vi "SmartInsert.vi"(8 "error in (no error)":errorcluster, 10 "VI reference In":refnum<vi>, 11 "SelList[]":refnum<vi>[](array[refnum])) -> (0 "error out":errorcluster)   [LabVIEW 2014]
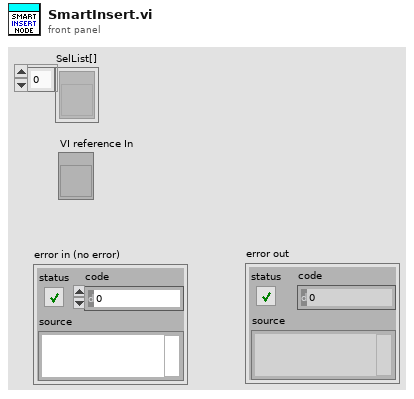
[diagram p1: front panel]
types:
  T1 = cluster{"Source":refnum<vi>, "Sink":refnum<vi>, "Type Variant":variant}
  T2 = typedef "LVPositionTypeDef.ctl" = cluster{"Left":i32, "Top":i32}
  T3 = cluster{"Position":cluster{"h":i16, "v":i16}, "Flags":i32, "Type":enum32{"LooseEnd", "Endpoint", "Bend", "Junction"}, "Up Joint Index":i16, "Down Joint Index":i16, "Left Joint Index":i16, "Right Joint Index":i16}[]
  T4 = typedef "LVPointTypeDef.ctl" = cluster{"Horizontal":i16, "Vertical":i16}
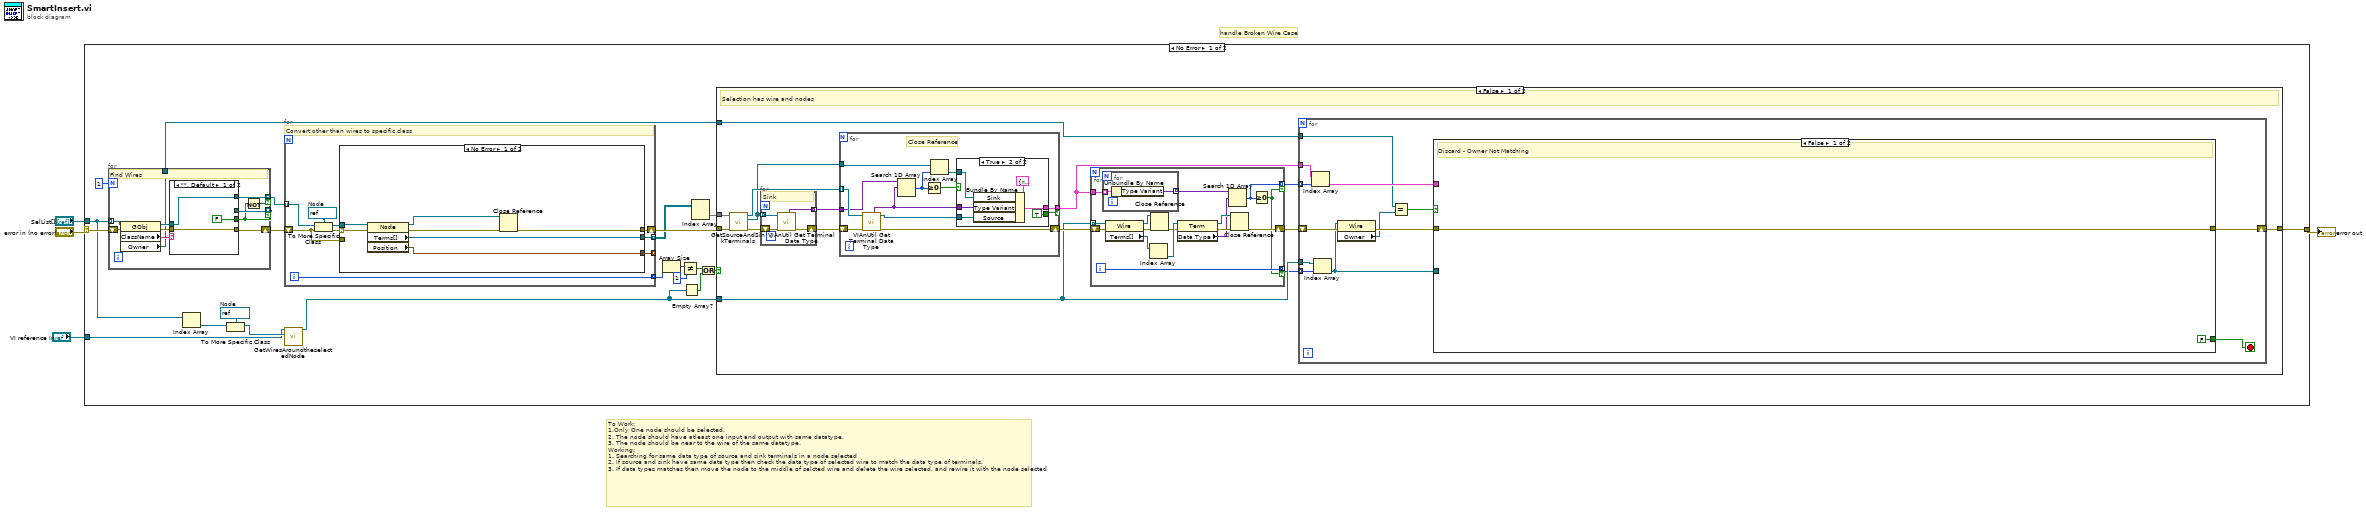
[diagram p0: block diagram]
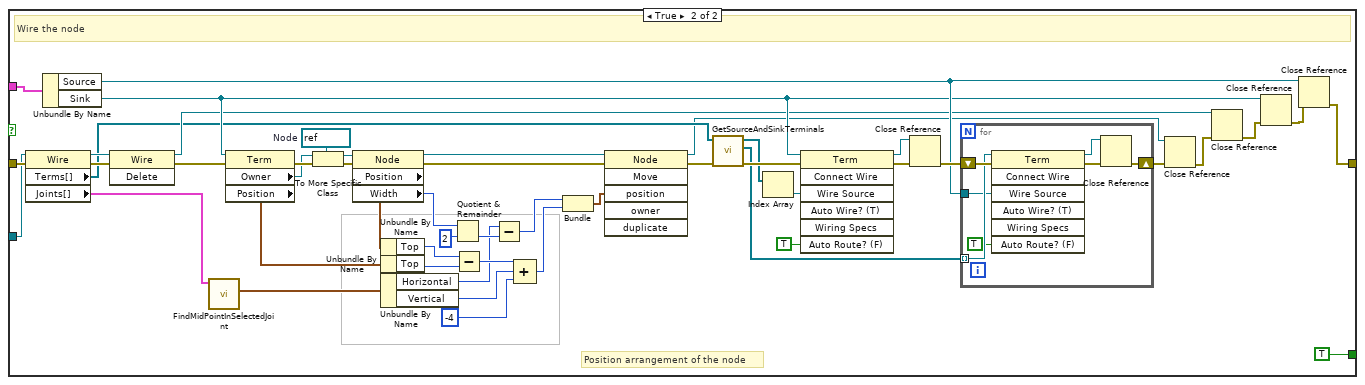
[diagram p2: hidden frame]
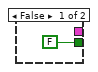
[diagram p3: hidden frame]
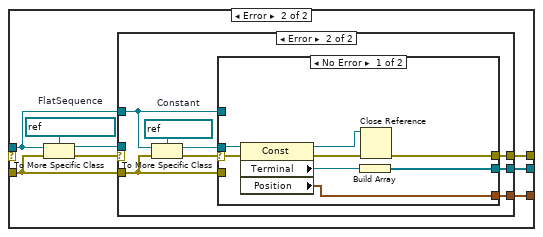
[diagram p5: hidden frame]
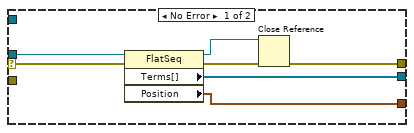
[diagram p6: hidden frame]
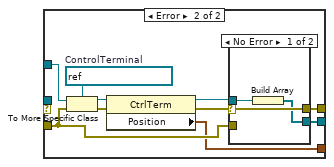
[diagram p7: hidden frame]
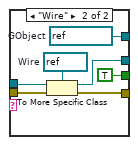
[diagram p9: hidden frame]
diagram:
  # "To Work:\n1.Only One node should be selected.\n2. The node should have atleast one input and output with same datatype.\n3. The node should be near to the wire of the same datatype.\nWorking:\n1. Searching for same data type of source and sink terminals in a node selected\n2. If source and sink have same data type then check the data type of selected wire to match the data type of terminals.\n3. If data types matches then move the node to the middle of selcted wire and delete the wire selected, and rewire it with the node selected"
  # "handle Broken Wire Case"
  n1 = case shown="No Error" "error in (no error)" {
    selector: "error in (no error)" -> [w25 w236]
    tunnel: [w21 w236] -> w2
    tunnel: "SelList[]" -> [w11 _]
    tunnel: "VI reference In" -> [w8 _]
    frame No Error {
      w12 = refnum<vi> refnum  # Node
      n2 = for {
        N: 1 -> [_]
        tunnel: w11 -> [w225] mode=indexing
        tunnel: [w219] -> _ mode=indexing if=w217
        shift-right: [w220] -> w24
        shift-left: w25 -> [w222]
        tunnel: [w218] -> w23 mode=indexing if=w216
        tunnel: [w215] -> w5
        # "Find Wires"
        n3 = property on="Property Node" class="GObj"(reference=w225, error in=w222) -> (reference out=w223:refnum<vi>, error out=w221:errorcluster, "ClassName"=w224:string, "Owner"=w215:refnum<vi>)
        n4 = case shown="\"\", Default" w224 {
          tunnel: w223 -> [w226 w233]
          tunnel: w221 -> [w227 w235]
          tunnel: [w227 w234] -> w220
          tunnel: [_ w231] -> w219
          tunnel: [FALSE TRUE] -> w217
          tunnel: [w226 w229] -> w218
          frame "", Default {
          }
          frame "Wire" {
            w229 = refnum<vi> refnum  # GObject
            w232 = refnum<vi> refnum  # Wire
            n5 = To More Specific Class(target class=w232, reference=w233, error in=w235) -> (specific class reference=w231:refnum<vi>, error out=w234:errorcluster)
          }
        }
        n6 = Not(x=w217) -> (.not. x?=w216:bool)
      }
      n7 = Index Array(array=w11) -> (element=w10:refnum<vi>)  [unwired: 1 in]
      n8 = To More Specific Class(target class=w12, reference=w10) -> (specific class reference=w9:refnum<vi>)  [unwired: 1 in, 1 out]
      n9 = for {
        tunnel: [w160] -> w20 mode=indexing
        shift-right: [w157] -> w22
        shift-left: w24 -> [w158]
        tunnel: w23 -> [w156] mode=indexing
        tunnel: [w155] -> w17 mode=indexing
        tunnel: [w154] -> _ mode=indexing
        i -> [w155]
        w159 = refnum<vi> refnum  # Node
        # "Convert other than wires to specific class"
        n10 = To More Specific Class(target class=w159, reference=w156, error in=w158) -> (specific class reference=w161:refnum<vi>, error out=w162:errorcluster)
        n11 = case shown="No Error" w162 {
          selector: w162 -> [w169 _]
          tunnel: w161 -> [w168 w171]
          tunnel: [w167 w173] -> w160
          tunnel: [w165 w175] -> w157
          tunnel: w158 -> [_ w174]
          tunnel: [w163 w170] -> w154
          frame No Error {
            n12 = property on="Property Node" class="Node"(reference=w168, error in=w169) -> (reference out=w164:refnum<vi>, error out=w166:errorcluster, "Terms[]"=w167:refnum<vi>[], "Position"=w163:T2)
            n13 = Close Reference(reference=w164, error in (no error)=w166) -> (error out=w165:errorcluster)
          }
          frame Error {
            w172 = refnum<vi> refnum  # FlatSequence
            n14 = To More Specific Class(target class=w172, reference=w171, error in=w174) -> (specific class reference=w176:refnum<vi>, error out=w177:errorcluster)
            n15 = case shown="Error" w177 {
              selector: w177 -> [w184 _]
              tunnel: w176 -> [w183 _]
              tunnel: [w180 w187] -> w175
              tunnel: w174 -> [_ w189]
              tunnel: [w181 w188] -> w173
              tunnel: w171 -> [_ w190]
              tunnel: [w178 w185] -> w170
              frame No Error {
                n16 = property on="Property Node" class="FlatSeq"(reference=w183, error in=w184) -> (reference out=w179:refnum<vi>, error out=w182:errorcluster, "Terms[]"=w181:refnum<vi>[], "Position"=w178:T2)
                n17 = Close Reference(reference=w179, error in (no error)=w182) -> (error out=w180:errorcluster)
              }
              frame Error {
                w186 = refnum<vi> refnum  # Constant
                n18 = To More Specific Class(target class=w186, reference=w190, error in=w189) -> (specific class reference=w191:refnum<vi>, error out=w192:errorcluster)
                n19 = case shown="No Error" w192 {
                  selector: w192 -> [w199 _]
                  tunnel: w191 -> [w200 _]
                  tunnel: w190 -> [_ w210]
                  tunnel: w189 -> [_ w208]
                  tunnel: [w197 w206] -> w188
                  tunnel: [w195 w207] -> w187
                  tunnel: [w193 w201] -> w185
                  frame No Error {
                    n20 = property on="Property Node" class="Const"(reference=w200, error in=w199) -> (reference out=w194:refnum<vi>, error out=w196:errorcluster, "Terminal"=w198:refnum<vi>, "Position"=w193:T2)
                    n21 = Build Array(w198) -> (w197:refnum<vi>[])
                    n22 = Close Reference(reference=w194, error in (no error)=w196) -> (error out=w195:errorcluster)
                  }
                  frame Error {
                    w205 = refnum<vi> refnum  # ControlTerminal
                    n23 = To More Specific Class(target class=w205, reference=w210, error in=w208) -> (specific class reference=w203:refnum<vi>, error out=w209:errorcluster)
                    n24 = property class="CtrlTerm"(reference=w203, error in=w209) -> (reference out=w202:refnum<vi>, error out=w204:errorcluster, "Position"=w201:T2)
                    n25 = case shown="No Error" w204 {
                      selector: w204 -> [w213 _]
                      tunnel: w202 -> [w212 _]
                      tunnel: w208 -> [_ w214]
                      tunnel: [w213 w214] -> w207
                      tunnel: [w211 _] -> w206
                      frame No Error {
                        n26 = Build Array(w212) -> (w211:refnum<vi>[])
                      }
                      frame Error {
                      }
                    }
                  }
                }
              }
            }
          }
        }
      }
      n27 = call "GetWiresAroundtheselectedNode.vi"("Sel Node reference"=w9, "VI reference In"=w8) -> ("WiresInRange[]"=w7:refnum<vi>[])  [unwired: 8 in, 1 out]
      n28 = Array Size(array=w17) -> (size(s)=w19:i32)
      n29 = Not Equal?(x=w19, y=1) -> (x != y?=w15:bool)
      n30 = Empty Array?(array=w7) -> (empty?=w14:bool)
      n31 = Index Array(array=w20) -> (element=w18:refnum<vi>[])  [unwired: 2 in]
      n32 = Or(x=w15, y=w14) -> (x .or. y?=w13:bool)
      n33 = case shown="False" w13 {
        tunnel: w7 -> [w32 _]
        tunnel: [w34 w153] -> w21
        tunnel: w22 -> [w40 w153]
        tunnel: w18 -> [w27 _]
        tunnel: w5 -> [w26 _]
        frame False {
          # "Selection has wire and nodes"
          n34 = call "GetSourceAndSinkTerminals.vi"("error in (no error)"=w40, "Terms[]"=w27) -> ("error out"=w38:errorcluster, "Sink"=w28:refnum<vi>[], "Source"=w36:refnum<vi>[])  [unwired: 7 in]
          n35 = for {
            tunnel: w28 -> [w133] mode=indexing
            tunnel: [w132] -> w39 mode=indexing
            shift-right: [w130] -> w37
            shift-left: w38 -> [w131]
            # "Sink"
            n36 = call <vilib>:"VIAnUtil Get Terminal Data Type.vi"("error in (no error)"=w131, "Terminal"=w133) -> ("error out"=w130:errorcluster, "Type Variant"=w132:variant)  [unwired: 6 in, 2 out]
          }
          n37 = for {
            tunnel: w39 -> [w144]
            tunnel: w36 -> [w145] mode=indexing
            shift-right: [w141] -> w35
            shift-left: w37 -> [w142]
            tunnel: w28 -> [w138]
            tunnel: [w135] -> w30 mode=indexing if=w134
            # "Close Reference"
            n38 = call <vilib>:"VIAnUtil Get Terminal Data Type.vi"("error in (no error)"=w142, "Terminal"=w145) -> ("error out"=w141:errorcluster, "dup  Terminal"=w140:refnum<vi>, "Type Variant"=w143:variant)  [unwired: 6 in, 1 out]
            n39 = Search 1D Array(1D array=w144, element=w143) -> (index of element=w139:i32)  [unwired: 1 in]
            n40 = Greater Or Equal To 0?(x=w139) -> (x >= 0?=w136:bool)
            n41 = Index Array(array=w138, index=w139) -> (element=w137:refnum<vi>)
            n42 = case shown="True" w136 {
              tunnel: w143 -> [_ w151]
              tunnel: w140 -> [_ w150]
              tunnel: w137 -> [_ w149]
              tunnel: [_ w148] -> w135
              tunnel: [FALSE TRUE] -> w134
              frame False {
              }
              frame True {
                n43 = Bundle By Name(cluster=T1 {"Source"=refnum, "Sink"=refnum, "Type Variant"=variant}, "Sink"=w149, "Type Variant"=w151, "Source"=w150) -> (w148:T1)
              }
            }
          }
          n44 = for {
            tunnel: w32 -> [w125] mode=indexing
            shift-right: [w121] -> w33
            shift-left: w35 -> [w127]
            tunnel: w30 -> [w119]
            tunnel: [w116] -> w29 mode=indexing if=w112
            tunnel: [w115] -> w31 mode=indexing if=w112
            i -> [w115]
            n45 = for {
              tunnel: w119 -> [w129] mode=indexing
              tunnel: [w128] -> w118 mode=indexing
              n46 = Unbundle By Name(w129) -> ("Type Variant"=w128:variant)
            }
            n47 = property on="Property Node" class="Wire"(reference=w125, error in=w127) -> (reference out=w113:refnum<vi>, error out=w126:errorcluster, "Terms[]"=w124:refnum<vi>[])
            n48 = Index Array(array=w124) -> (element=w122:refnum<vi>)  [unwired: 1 in]
            n49 = Close Reference(reference=w113, error in (no error)=w126) -> (error out=w114:errorcluster)
            n50 = property on="Property Node" class="Term"(reference=w122, error in=w114) -> (reference out=w120:refnum<vi>, error out=w123:errorcluster, "Data Type"=w117:variant)
            n51 = Search 1D Array(1D array=w118, element=w117) -> (index of element=w116:i32)  [unwired: 1 in]
            n52 = Close Reference(reference=w120, error in (no error)=w123) -> (error out=w121:errorcluster)
            n53 = Greater Or Equal To 0?(x=w116) -> (x >= 0?=w112:bool)
          }
          n54 = for {
            tunnel: w32 -> [w51]
            tunnel: w31 -> [w50] mode=indexing
            tunnel: w30 -> [w49]
            tunnel: w29 -> [w47] mode=indexing
            shift-right: [w53] -> w34
            shift-left: w33 -> [w52]
            tunnel: w26 -> [w42]
            stop <- w46 stop-if-true
            n55 = Index Array(array=w49, index=w47) -> (element=w48:T1)
            n56 = Index Array(array=w51, index=w50) -> (element=w44:refnum<vi>)
            n57 = property class="Wire"(reference=w44, error in=w52) -> (error out=w45:errorcluster, "Owner"=w43:refnum<vi>)  [unwired: 1 out]
            n58 = Equal?(x=w42, y=w43) -> (x = y?=w41:bool)
            n59 = case shown="False" w41 {
              tunnel: [w55 w95] -> w53
              tunnel: w45 -> [w55 w104]
              tunnel: w48 -> [_ w58]
              tunnel: w44 -> [_ w57]
              tunnel: [FALSE TRUE] -> w46
              frame False {
                # "Discard - Owner Not Matching"
              }
              frame True {
                w87 = refnum<vi> refnum  # Node
                # "Position arrangement of the node"
                # "Wire the node"
                n60 = property on="Property Node" class="Wire"(reference=w57, error in=w104) -> (reference out=w91:refnum<vi>, error out=w103:errorcluster, "Terms[]"=w67:refnum<vi>[], "Joints[]"=w90:T3)
                n61 = Unbundle By Name(w58) -> ("Source"=w89:refnum<vi>, "Sink"=w69:refnum<vi>)
                n62 = invoke on="Invoke Node" class="Wire" method="Delete"(reference=w91, error in=w103) -> (reference out=w68:refnum<vi>, error out=w71:errorcluster)  [unwired: 1 in, 1 out]
                n63 = call "FindMidPointInSelectedJoint.vi"("Joints[]"=w90) -> ("MidPoint"=w64:T4)  [unwired: 8 in, 2 out]
                n64 = property on="Property Node" class="Term"(reference=w69, error in=w71) -> (error out=w86:errorcluster, "Owner"=w85:refnum<vi>, "Position"=w83:T2)  [unwired: 1 out]
                n65 = To More Specific Class(target class=w87, reference=w85, error in=w86) -> (specific class reference=w76:refnum<vi>, error out=w75:errorcluster)
                n66 = property on="Property Node" class="Node"(reference=w76, error in=w75) -> (reference out=w74:refnum<vi>, error out=w73:errorcluster, "Position"=w84:T2, "Width"=w78:u32)
                n67 = Unbundle By Name(w84) -> ("Top"=w82:i32)
                n68 = Unbundle By Name(w83) -> ("Top"=w81:i32)
                n69 = Unbundle By Name(w64) -> ("Horizontal"=w63:i16, "Vertical"=w62:i16)
                n70 = Quotient & Remainder(x=w78, y=u32 2) -> (floor(x/y)=w79:u32)  [unwired: 1 out]
                n71 = Subtract(x=w82, y=w81) -> (x-y=w80:i32)
                n72 = Subtract(x=w63, y=w79) -> (x-y=w61:u32)
                n73 = Compound Arithmetic op=ADD(w80, w62, i16 -4 ("value")) -> (w60:i32)
                n74 = Bundle(w61, w60) -> (w59:cluster{u32, i32})  [unwired: 1 in]
                n75 = invoke on="Invoke Node" class="Node" method="Move"(reference=w74, error in=w73, "position"=w59) -> (reference out=w65:refnum<vi>, error out=w70:errorcluster)  [unwired: 3 in, 4 out]
                n76 = call "GetSourceAndSinkTerminals.vi"("error in (no error)"=w70, "Terms[]"=w67) -> ("error out"=w102:errorcluster, "Sink"=w98:refnum<vi>[], "Source"=w101:refnum<vi>[])  [unwired: 7 in]
                n77 = Index Array(array=w101) -> (element=w100:refnum<vi>)  [unwired: 1 in]
                n78 = invoke on="Invoke Node" class="Term" method="Connect Wire"(reference=w69, error in=w102, "Wire Source"=w100, "Auto Route? (F)"=TRUE) -> (reference out=w93:refnum<vi>, error out=w99:errorcluster)  [unwired: 3 in, 5 out]
                n79 = Close Reference(reference=w93, error in (no error)=w99) -> (error out=w94:errorcluster)
                n80 = for {
                  shift-right: [w107] -> w66
                  shift-left: w94 -> [w111]
                  tunnel: w98 -> [w109] mode=indexing
                  tunnel: w89 -> [w108]
                  n81 = invoke on="Invoke Node" class="Term" method="Connect Wire"(reference=w109, error in=w111, "Wire Source"=w108, "Auto Route? (F)"=TRUE) -> (reference out=w106:refnum<vi>, error out=w110:errorcluster)  [unwired: 3 in, 5 out]
                  n82 = Close Reference(reference=w106, error in (no error)=w110) -> (error out=w107:errorcluster)
                }
                n83 = Close Reference(reference=w65, error in (no error)=w66) -> (error out=w88:errorcluster)
                n84 = Close Reference(reference=w68, error in (no error)=w88) -> (error out=w97:errorcluster)
                n85 = Close Reference(reference=w69, error in (no error)=w97) -> (error out=w96:errorcluster)
                n86 = Close Reference(reference=w89, error in (no error)=w96) -> (error out=w95:errorcluster)
              }
            }
          }
        }
        frame True {
          # "No Nodes or Wires in selection. Discard"
        }
      }
    }
    frame Error {
    }
  }
  "error out" <- w2
